vi "Draw Stats.vi"(10 "Stats":T1={"Transform And Project Duration"=0.0, "Raster Duration"=0.0, "Present Duration"=82.5692473, "Frame Rate"=111.70812900055276, "Visible Triangles"=0, "Delta Time"=0.0} {"Delta Time" format="%.0p"; "Frame Rate" format="%.0p"; "Present Duration" format="%.0p"; "Raster Duration" format="%.0p"; "Transform And Project Duration" format="%.0p"}, 11 "Screen in":picture) -> (3 "Screen out":picture)   [LabVIEW 2020, in "Example 1.lvlib"]
uses:
  Example 1.lvlib
  Graphics/Libraries/Utility/Utility.lvlib
  Scene/Stats.ctl
  Scene/Scene.lvclass
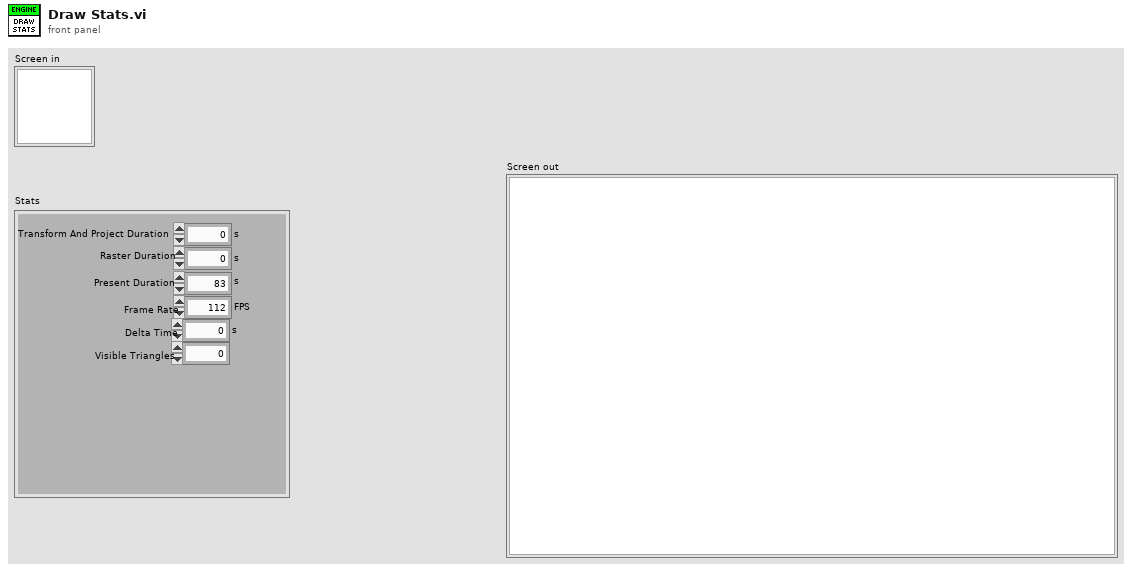
[diagram p1: front panel]
types:
  T1 = typedef "Scene.lvclass/Stats.ctl" = cluster{"Transform And Project Duration":dbl, "Raster Duration":dbl, "Present Duration":dbl, "Frame Rate":dbl, "Visible Triangles":i32, "Delta Time":dbl}
  T2 = enum16{"User-specified Font", "Application Font", "System Font", "Dialog Font"}
  T3 = cluster{"Font Name:":string, "Size":i16, "Strikeout?":bool, "Italic?":bool, "Underline?":bool, "Outline?":bool, "Shadow?":bool, "Bold?":bool}
  T4 = cluster{"left":i16, "top":i16, "right":i16, "bottom":i16}
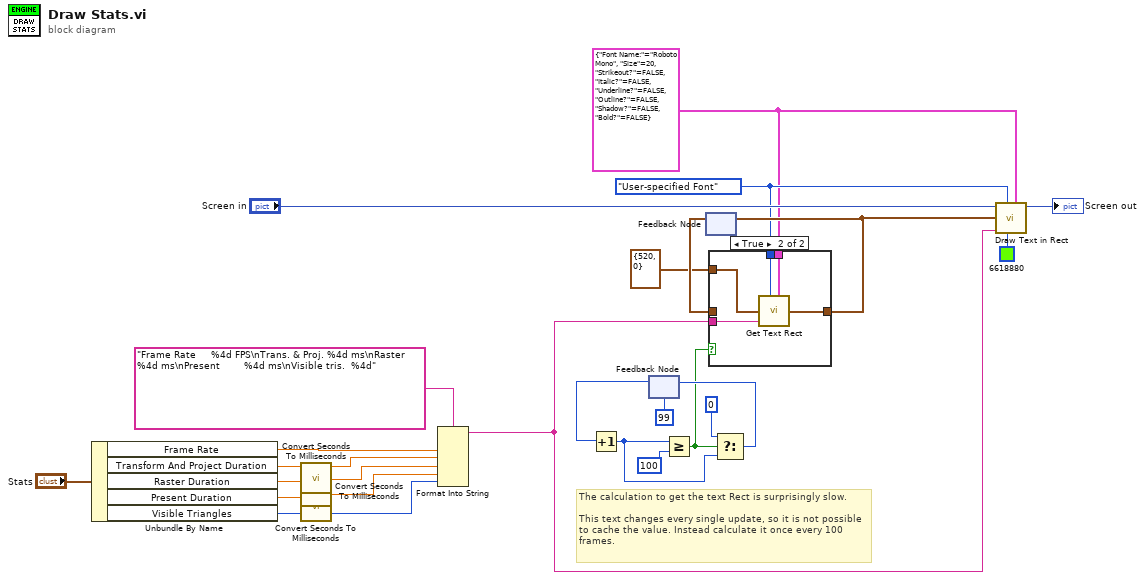
[diagram p0: block diagram]
diagram:
  w10 = T2."User-specified Font" ("desired font(Application)")
  w9 = T3 {"Font Name:"="Roboto Mono", "Size"=20, "Strikeout?"=FALSE, "Italic?"=FALSE, "Underline?"=FALSE, "Outline?"=FALSE, "Shadow?"=FALSE, "Bold?"=FALSE} ("[user-specified font]")
  # "The calculation to get the text Rect is surprisingly slow.\n\nThis text changes every single update, so it is not possible to cache the value. Instead calculate it once every 100 frames."
  n1 = Unbundle By Name("Stats") -> ("Frame Rate"=w21:dbl, "Transform And Project Duration"=w19:dbl, "Raster Duration"=w17:dbl, "Present Duration"=w15:dbl, "Visible Triangles"=w20:i32)
  n2 = call "Convert Seconds To Milliseconds.vi"("Seconds"=w19) -> ("Milliseconds"=w18:dbl)  [unwired: 10 in]
  n3 = call "Convert Seconds To Milliseconds.vi"("Seconds"=w17) -> ("Milliseconds"=w16:dbl)  [unwired: 10 in]
  n4 = call "Convert Seconds To Milliseconds.vi"("Seconds"=w15) -> ("Milliseconds"=w14:dbl)  [unwired: 10 in]
  n5 = Format Into String(format string="Frame Rate     %4d FPS\nTrans. & Proj. %4d ms\nRaster         %4d ms\nPresent        %4d ms\nVisible tris.  %4d", w21, w18, w16, w14, w20) -> (resulting string=w8:string)  [unwired: 2 in, 1 out]
  n6 = feedback #1(u32 99) -> (w7:u32)
  n7 = Increment(x=w7) -> (x+1=w2:u32)
  n8 = Greater Or Equal?(x=w2, y=u32 100) -> (x >= y?=w1:bool)
  n9 = feedback #2() -> (w12:T4)  [unwired: 1 in]
  n10 = case shown="True" w1 {
    tunnel: [w27 w32] -> w13
    tunnel: w12 -> [w27 _]
    tunnel: cluster{"x":i16, "y":i16} {"x"=520, "y"=0} ("origin") -> [_ w31]
    tunnel: w10 -> [_ w30]
    tunnel: w9 -> [_ w29]
    tunnel: w8 -> [_ w28]
    frame False {
    }
    frame True {
      n11 = call <vilib>:"Get Text Rect.vi"("desired font(Application)"=w30, "origin(0,0)"=w31, "text"=w28, "[user-specified font]"=w29) -> ("rect"=w32:T4)  [unwired: 5 in]
    }
  }
  n12 = feedback-in #2(w13) -> ()
  n13 = Select(t=u32 0 ("y"), s=w1, f=w2) -> (s? t:f=w3:u32)
  n14 = feedback-in #1(w3) -> ()
  n15 = call <vilib>:"Draw Text in Rect.vi"("[user-specified font]"=w9, "text color(black)"=u32 6618880, "desired font(Application)"=w10, "text"=w8, "rect"=w13, "picture"="Screen in") -> ("new picture"=→"Screen out":picture)  [unwired: 5 in]
